vi "MGCC_StaEst_test_output.vi"() -> ()   [LabVIEW 2016]
uses:
  <vilib>/Utility/file.llb/Write Delimited Spreadsheet (DBL).vi
panel:
  in  "Ve":dbl[][](array[numeric])
  in  "Vf":dbl[][](array[numeric])
  in  "VOL":cdb[][](array[numeric])
  in  "AN":dbl[][](array[numeric])
  in  "Vn":dbl[][](array[numeric])
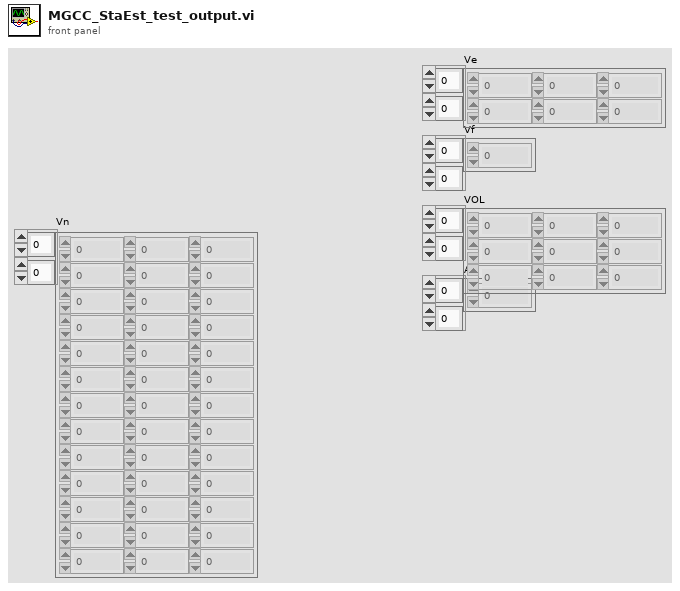
[diagram p1: front panel]
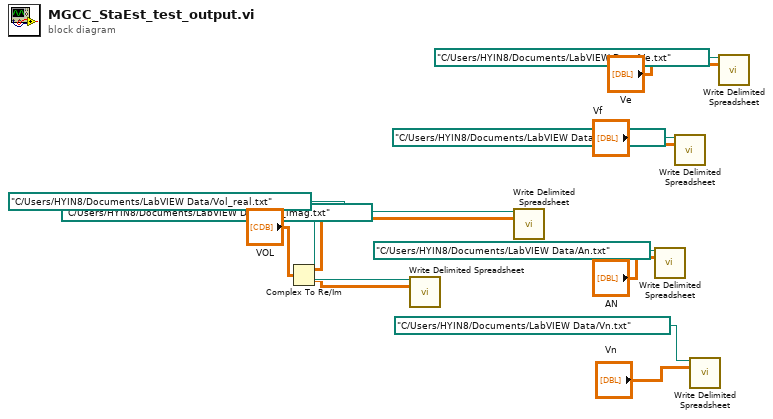
[diagram p0: block diagram]
diagram:
  n1 = Complex To Re/Im(x + iy="VOL") -> (x=w3:dbl[][], y=w1:dbl[][])
  n2 = call-poly <vilib>:"Write Delimited Spreadsheet.vi"("file path (dialog if empty)"=path "C:/Users/HYIN8/Documents/LabVIEW Data/Vol_imag.txt", "2D data"=w1) -> ()  [unwired: 12 in, 2 out]
  n3 = call-poly <vilib>:"Write Delimited Spreadsheet.vi"("file path (dialog if empty)"=path "C:/Users/HYIN8/Documents/LabVIEW Data/Vol_real.txt", "2D data"=w3) -> ()  [unwired: 12 in, 2 out]
  n4 = call-poly <vilib>:"Write Delimited Spreadsheet.vi"("file path (dialog if empty)"=path "C:/Users/HYIN8/Documents/LabVIEW Data/An.txt", "2D data"="AN") -> ()  [unwired: 12 in, 2 out]
  n5 = call-poly <vilib>:"Write Delimited Spreadsheet.vi"("file path (dialog if empty)"=path "C:/Users/HYIN8/Documents/LabVIEW Data/Vf.txt", "2D data"="Vf") -> ()  [unwired: 12 in, 2 out]
  n6 = call-poly <vilib>:"Write Delimited Spreadsheet.vi"("file path (dialog if empty)"=path "C:/Users/HYIN8/Documents/LabVIEW Data/Vn.txt", "2D data"="Vn") -> ()  [unwired: 12 in, 2 out]
  n7 = call-poly <vilib>:"Write Delimited Spreadsheet.vi"("file path (dialog if empty)"=path "C:/Users/HYIN8/Documents/LabVIEW Data/Ve.txt", "2D data"="Ve") -> ()  [unwired: 12 in, 2 out]
